vi "测试接收队列.vi"() -> ()   [LabVIEW 2015]
uses:
  <userlib>/QMH/Message Queue/Support/Enqueue Message (Single).vi
  <vilib>/Utility/error.llb/Error Cluster From Error Code.vi
  <vilib>/ErrorRing/Error Ring.xnode
  <userlib>/QMH/User Event - Stop/User Event - Stop.lvlib
  <userlib>/QMH/Message Queue/Message Queue.lvlib
panel:
  in  "表格":string[][](table)
  in  "Exit":bool
  in  "HostThread":variant
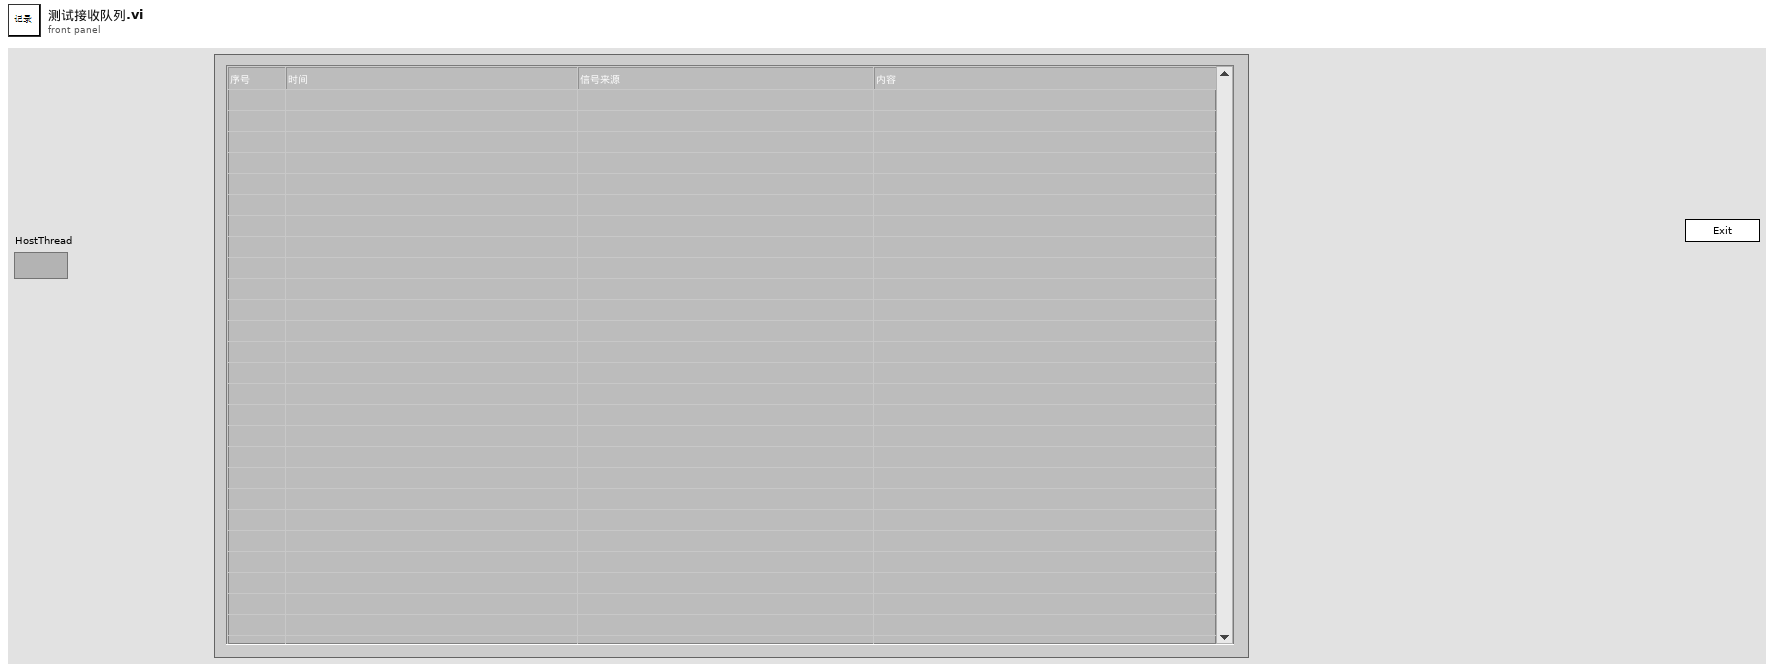
[diagram p1: front panel]
types:
  T1 = cluster{"Controls":cluster{"Exit":refnum<vi>, "表格":refnum<vi>}, "Thread":cluster{"ThisQ":string, "ThisVI":refnum<vi>, "HostQ":string, "HostRef":refnum<vi>, "SlavesQ":string[], "SlavesRef":refnum<vi>[]}, "Data":cluster{"Replace":bool}, "User":cluster{"Name":string}, "文本":string[], "计数":i32}
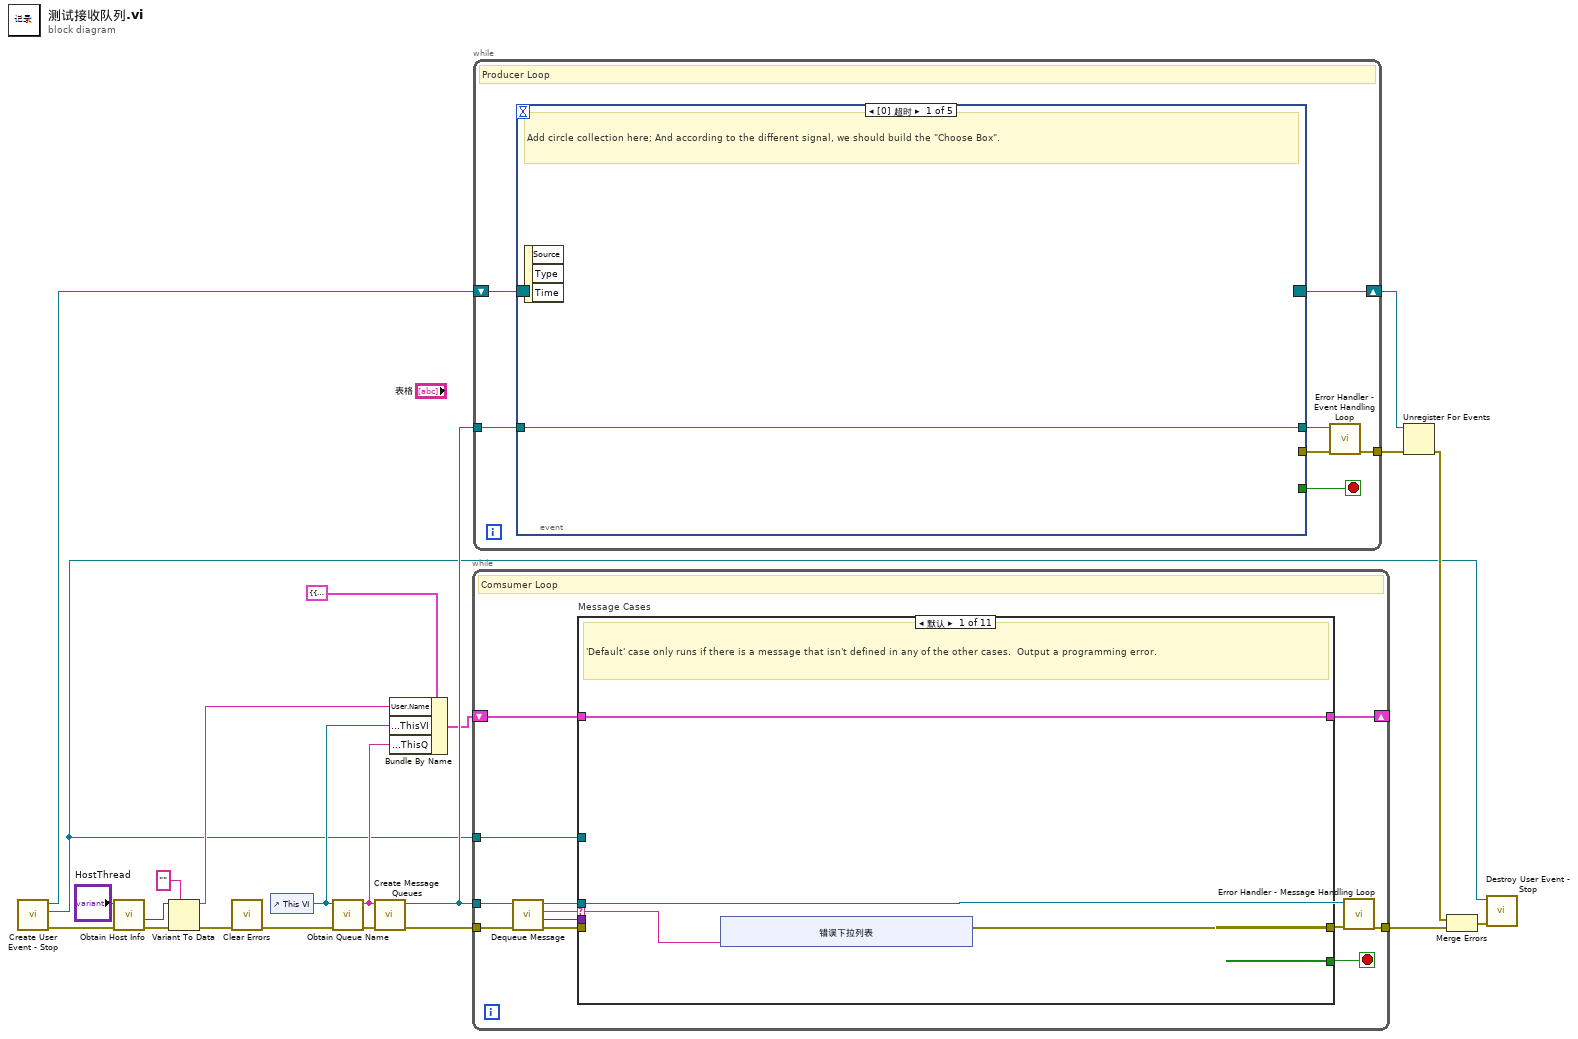
[diagram p0: block diagram]
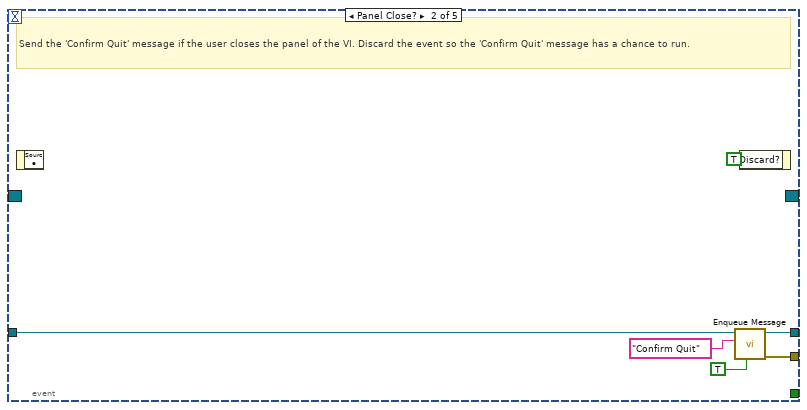
[diagram p2: hidden frame]
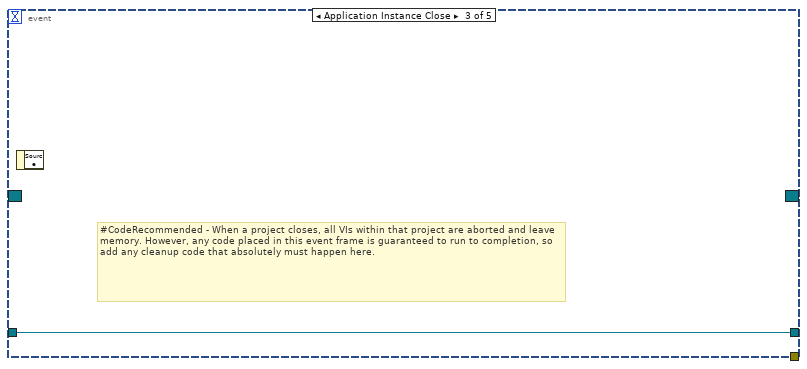
[diagram p3: hidden frame]
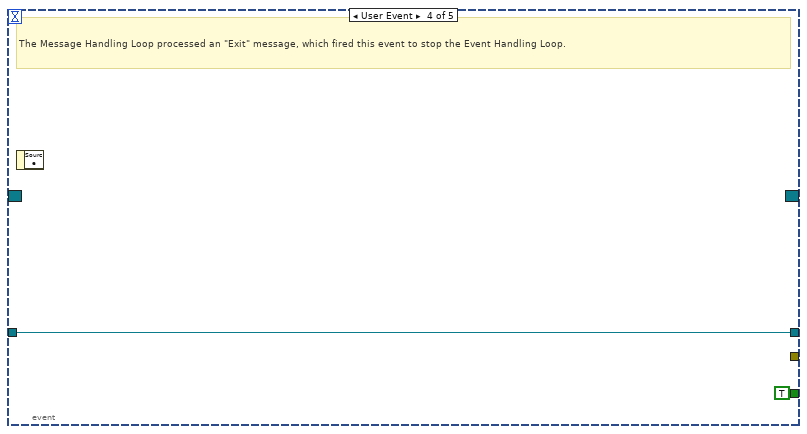
[diagram p4: hidden frame]
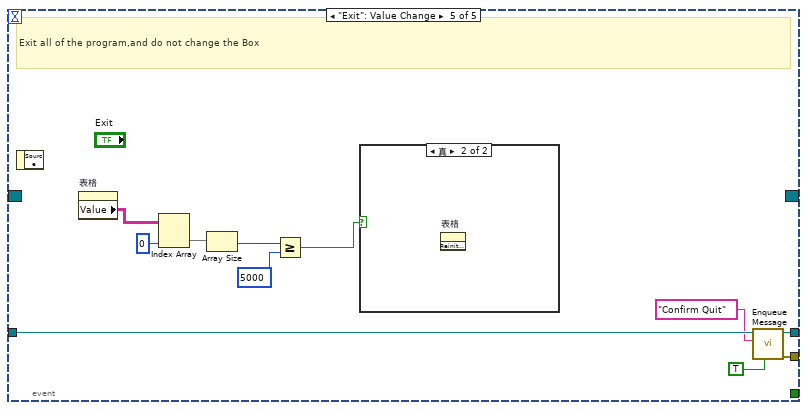
[diagram p5: hidden frame]
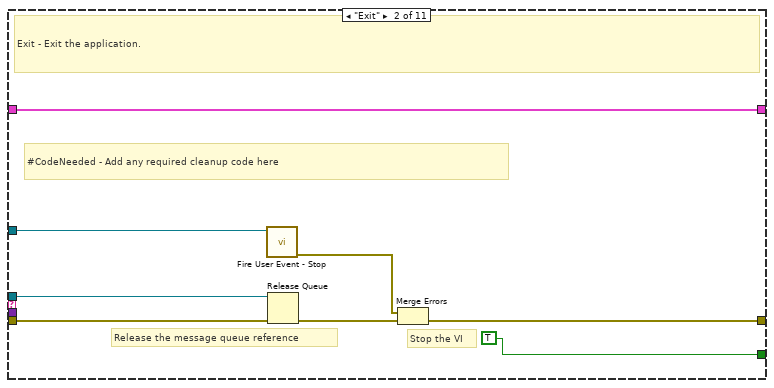
[diagram p7: hidden frame]
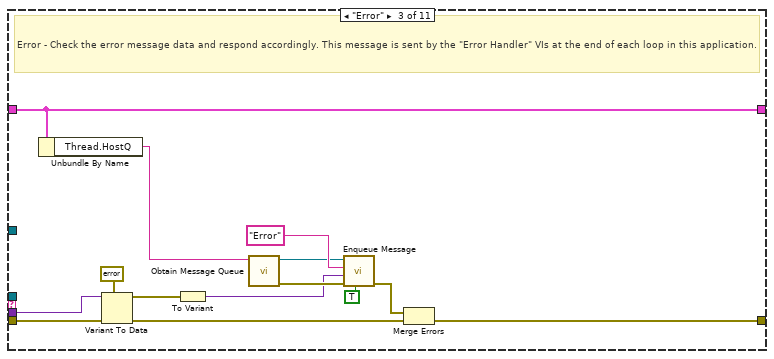
[diagram p8: hidden frame]
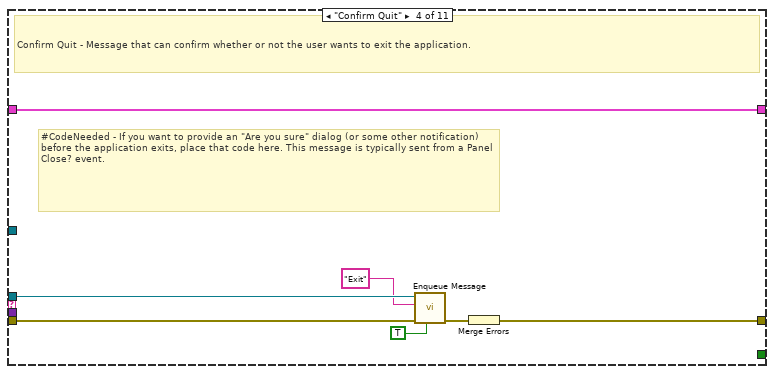
[diagram p9: hidden frame]
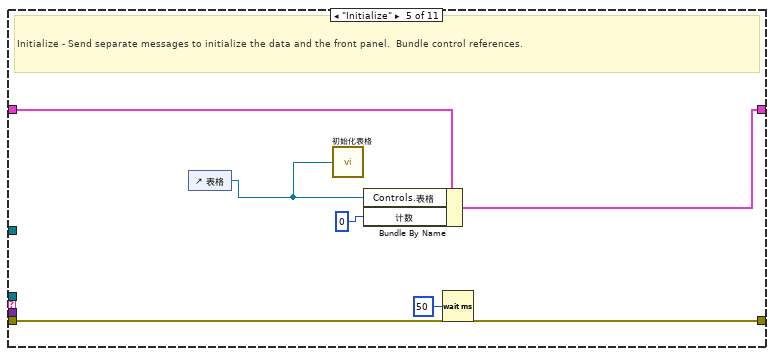
[diagram p10: hidden frame]
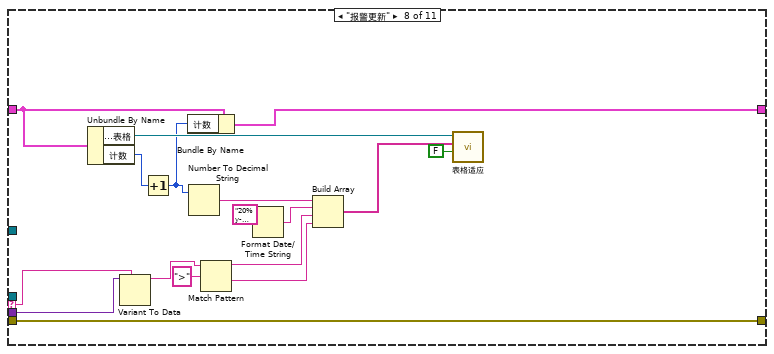
[diagram p13: hidden frame]
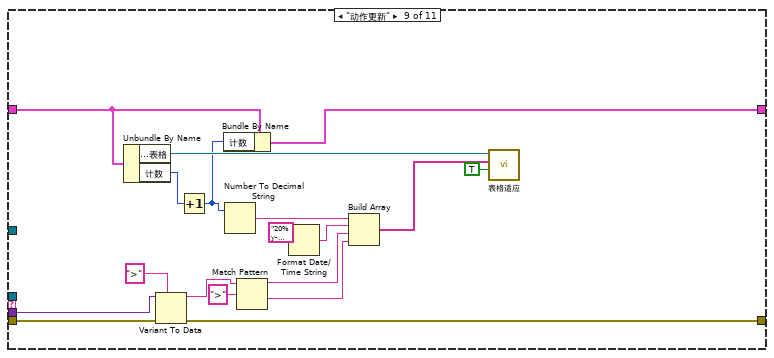
[diagram p14: hidden frame]
diagram:
  n1 = call <userlib>:"Create User Event - Stop.vi"() -> ("error out"=w14:errorcluster, "User Event - Stop"=w5:refnum<user-event>, "Stop Event Registration Refnum"=w3:refnum<event-registration>)  [unwired: 9 in]
  n2 = call <userlib>:"Obtain Host Info.vi"("error in (no error)"=w14, "HostThread"="HostThread") -> ("error out"=w17:errorcluster, "Data"=w18:variant)  [unwired: 6 in, 2 out]
  n3 = Variant To Data(error in=w17, type="", Variant=w18) -> (data=w22:string, error out=w20:errorcluster)
  n4 = call <vilib>:"Clear Errors.vi"("error in (no error)"=w20) -> ("error out"=w21:errorcluster)  [unwired: 5 in, 1 out]
  n5 = control-ref of="This VI"() -> (w12:refnum<vi>)
  n6 = call <userlib>:"Obtain Queue Name.vi"("error in (no error)"=w21, "VI Refnum"=w12) -> ("error out"=w9:errorcluster, "ViName"=w13:string)  [unwired: 8 in]
  n7 = call <userlib>:"Create Message Queues.vi"("error in (no error)"=w9, "name (unnamed)"=w13) -> ("error out"=w1:errorcluster, "QueueHandler"=w16:refnum<queue>)  [unwired: 8 in]
  n8 = Bundle By Name(cluster=T1 {"Controls"={"Exit"=refnum, "表格"=refnum}, "Thread"={"ThisQ"="", "ThisVI"=refnum, "HostQ"="", "HostRef"=refnum, "SlavesQ"=[], "SlavesRef"=[]}, "Data"={"Replace"=FALSE}, "User"={"Name"=""}, "文本"=[], "计数"=0} ("Data Cluster"), "User.Name"=w22, "Thread.ThisVI"=w12, "Thread.ThisQ"=w13) -> (w11:T1)
  n9 = while {
    tunnel: w16 -> [w26]
    shift-right: [w33] -> _
    shift-left: w11 -> [w34]
    tunnel: w5 -> [w31]
    tunnel: w1 -> [w30]
    tunnel: [w24] -> w2
    stop <- w32 stop-if-true
    # "Comsumer Loop"
    n10 = call <userlib>:"Dequeue Message.vi"("error in (no error)"=w30, "Message Queue"=w26) -> ("error out"=w29:errorcluster, "Message Data"=w27:variant, "Message"=w28:string, "dup Message Queue"=w25:refnum<queue>)  [unwired: 6 in]
    n11 = case "Message Cases" shown="默认" w28 {
      selector: w28 -> [w35 _ _ _ _ _ _ w98 _ _ _]
      tunnel: w25 -> [_ w52 _ w69 _ _ _ _ _ _ _]
      tunnel: w29 -> [_ w47 w66 w73 w79 w81 w83 w100 w117 w118 w121]
      tunnel: [w36 w48 w61 w71 w79 w81 w83 w100 w117 w118 w121] -> w23
      tunnel: w34 -> [w37 w51 w58 w72 w78 w80 w82 w86 w104 w119 w120]
      tunnel: [w37 w51 w58 w72 w77 w80 w82 w85 w105 w119 w120] -> w33
      tunnel: [_ TRUE _ _ _ _ _ _ _ _ _] -> w32
      tunnel: w27 -> [_ _ w65 _ _ _ _ w99 w103 _ _]
      tunnel: w31 -> [_ w46 _ _ _ _ _ _ _ _ _]
      frame Default {
        # "'Default' case only runs if there is a message that isn't defined in any of the other cases.  Output a programming error."
        n12 = xnode "错误下拉列表"("参数 0"=w35) -> ("错误输出"=w36:errorcluster)
      }
      frame "Exit" {
        # "Stop the VI"
        # "Release the message queue reference"
        # "#CodeNeeded - Add any required cleanup code here"
        # "Exit - Exit the application."
        n13 = call <userlib>:"Fire User Event - Stop.vi"("User Event - Stop"=w46) -> ("error out"=w45:errorcluster)  [unwired: 10 in]
        n14 = Release Queue(queue=w52, error in (no error)=w47) -> (error out=w49:errorcluster)  [unwired: 1 in, 2 out]
        n15 = Merge Errors(w45, w49) -> (w48:errorcluster)
      }
      frame "Error" {
        # "Error - Check the error message data and respond accordingly. This message is sent by the \"Error Handler\" VIs at the end of each loop in this application."
        n16 = Unbundle By Name(w58) -> ("Thread.HostQ"=w57:string)
        n17 = Variant To Data(error in=w66, type=errorcluster {"status"=FALSE, "code"=0, "source"=""} ("error constant"), Variant=w65) -> (data=w54:errorcluster, error out=w63:errorcluster)
        n18 = To Variant(anything=w54) -> (Variant=w53:variant)
        n19 = call <userlib>:"Obtain Message Queue.vi"("name (unnamed)"=w57) -> ("error out"=w56:errorcluster, "Message Queue"=w55:refnum<queue>)  [unwired: 9 in]
        n20 = call-poly <userlib>:"Enqueue Message.vi"("Priority Message? (F)"=TRUE, "error in (no error)"=w56, "Message Data"=w53, "Message"="Error", "Message Queue"=w55) -> ("error out"=w62:errorcluster)  [unwired: 5 in, 1 out]
        n21 = Merge Errors(w62, w63) -> (w61:errorcluster)
      }
      frame "Confirm Quit" {
        # "#CodeNeeded - If you want to provide an \"Are you sure\" dialog (or some other notification) before the application exits, place that code here. This message is typically sent from a Panel Close? event."
        # "Confirm Quit - Message that can confirm whether or not the user wants to exit the application."
        n22 = call-poly <userlib>:"Enqueue Message.vi"("Priority Message? (F)"=TRUE, "error in (no error)"=w73, "Message"="Exit", "Message Queue"=w69) -> ("error out"=w70:errorcluster)  [unwired: 6 in, 1 out]
        n23 = Merge Errors(w70) -> (w71:errorcluster)
      }
      frame "Initialize" {
        # "Initialize - Send separate messages to initialize the data and the front panel.  Bundle control references."
        n24 = control-ref of="表格"() -> (w74:refnum<vi>)
        n25 = call "初始化表格.vi"("引用"=w74) -> ()
        n26 = Bundle By Name(cluster=w78, "Controls.表格"=w74, "计数"=0) -> (w77:T1)
        n27 = Wait (ms)(milliseconds to wait=u32 50 ("等待时间（毫秒）")) -> ()  [unwired: 1 out]
      }
      frame "<-------UI-------->" {
      }
      frame "<------Core------>" {
      }
      frame "报警更新" {
        n28 = Unbundle By Name(w86) -> ("Controls.表格"=w90:refnum<vi>, "计数"=w96:i32)
        n29 = Variant To Data(type=w98, Variant=w99) -> (data=w97:string)  [unwired: 1 in, 1 out]
        n30 = Increment(x=w96) -> (x+1=w84:i32)
        n31 = Bundle By Name(cluster=w86, "计数"=w84) -> (w85:T1)
        n32 = Number To Decimal String(number=w84) -> (decimal integer string=w95:string)  [unwired: 1 in]
        n33 = Match Pattern(string=w97, regular expression=">" ("正则表达式")) -> (before substring=w92:string, after substring=w91:string)  [unwired: 1 in, 2 out]
        n34 = Format Date/Time String(time format string (%c)="20%y-%m-%d  %H：%M：%S" ("时间格式字符串(%c)")) -> (date/time string=w93:string)  [unwired: 2 in]
        n35 = Build Array(w95, w93, w92, w91) -> (w89:string[])
        n36 = call "表格适应.vi"("Red-F"=FALSE, "new"=w89, "表格in"=w90) -> ()  [unwired: 9 in]
      }
      frame "动作更新" {
        n37 = Unbundle By Name(w104) -> ("Controls.表格"=w110:refnum<vi>, "计数"=w116:i32)
        n38 = Variant To Data(type=">" ("正则表达式"), Variant=w103) -> (data=w101:string)  [unwired: 1 in, 1 out]
        n39 = Increment(x=w116) -> (x+1=w106:i32)
        n40 = Bundle By Name(cluster=w104, "计数"=w106) -> (w105:T1)
        n41 = Number To Decimal String(number=w106) -> (decimal integer string=w115:string)  [unwired: 1 in]
        n42 = Match Pattern(string=w101, regular expression=">" ("正则表达式")) -> (before substring=w112:string, after substring=w111:string)  [unwired: 1 in, 2 out]
        n43 = Format Date/Time String(time format string (%c)="20%y-%m-%d  %H：%M：%S" ("时间格式字符串(%c)")) -> (date/time string=w113:string)  [unwired: 2 in]
        n44 = Build Array(w115, w113, w112, w111) -> (w109:string[])
        n45 = call "表格适应.vi"("Red-F"=TRUE, "new"=w109, "表格in"=w110) -> ()  [unwired: 9 in]
      }
      frame "Core_InitializeRef" {
        # "Initialize control references. For there is not enough space to locate all the control references, separate the codes into 2 messages"
      }
      frame "<---Operation--->" {
      }
    }
    n46 = call <userlib>:"Error Handler - Message Handling Loop.vi"("error in (no error)"=w23, "Message Queue"=w25) -> ("dup error in"=w24:errorcluster)  [unwired: 8 in, 1 out]
  }
  n47 = while {
    tunnel: w16 -> [w128]
    shift-right: [w126] -> w7
    shift-left: w3 -> [w127]
    tunnel: [w122] -> w8
    stop <- w124 stop-if-true
    # "Producer Loop"
    n48 = event shown="[0] 超时" {
      selector: w127 -> [_ _ _ _ _]
      dyn-events: [_ _ _ _ _] -> w126
      timeout: _ -> [_ _ _ _ _]
      tunnel: [_ _ _ TRUE ("Discard?") _] -> w124
      tunnel: w128 -> [w129 w134 w136 w138 w149]
      tunnel: [_ w133 _ _ w147] -> w125
      tunnel: [w129 w132 w136 w138 w148] -> w123
      event Timeout {
        # "Add circle collection here; And according to the different signal, we should build the \"Choose Box\"."
        n49 = event-data() -> ()  [unwired: 1 in, 3 out]
      }
      event Panel Close? {
        # "Send the 'Confirm Quit' message if the user closes the panel of the VI. Discard the event so the 'Confirm Quit' message has a chance to run."
        n50 = event-data() -> ()  [unwired: 1 in, 1 out]
        n51 = call-poly <userlib>:"Enqueue Message.vi"("Priority Message? (F)"=TRUE, "Message"="Confirm Quit", "Message Queue"=w134) -> ("error out"=w133:errorcluster, "dup Message Queue"=w132:refnum<queue>)  [unwired: 7 in]
        n52 = event-data("Discard?"=TRUE) -> ()  [unwired: 1 in, 1 out]
      }
      event Application Instance Close {
        # "#CodeRecommended - When a project closes, all VIs within that project are aborted and leave memory. However, any code placed in this event frame is guaranteed to run to completion, so add any cleanup code that absolutely must happen here."
        n53 = event-data() -> ()  [unwired: 1 in, 1 out]
      }
      event User Event {
        # "The Message Handling Loop processed an \"Exit\" message, which fired this event to stop the Event Handling Loop."
        n54 = event-data() -> ()  [unwired: 1 in, 1 out]
      }
      event "Exit": Value Change {
        # "Exit all of the program,and do not change the Box"
        n55 = event-data() -> ()  [unwired: 1 in, 1 out]
        n56 = property on="表格" class="Tbl (严格)"() -> ("Value"=w142:string[][])  [unwired: 2 in, 2 out]
        n57 = Index Array(array=w142, index (col)=0 ("禁用的索引 (列)")) -> (element=w143:string[])  [unwired: 1 in]
        n58 = Array Size(array=w143) -> (size(s)=w141:i32)
        n59 = Greater Or Equal?(x=w141, y=5000) -> (x >= y?=w139:bool)
        n60 = case shown="真" w139 {
          frame False {
          }
          frame True {
            n61 = invoke on="表格" class="Tbl (严格)" method="Reinit To Default"() -> ()  [unwired: 3 in, 3 out]
          }
        }
        n62 = call-poly <userlib>:"Enqueue Message.vi"("Priority Message? (F)"=TRUE, "Message"="Confirm Quit", "Message Queue"=w149) -> ("error out"=w147:errorcluster, "dup Message Queue"=w148:refnum<queue>)  [unwired: 7 in]
      }
    }
    n63 = call <userlib>:"Error Handler - Event Handling Loop.vi"("error in (no error)"=w125, "Message Queue"=w123) -> ("dup error in"=w122:errorcluster)  [unwired: 8 in, 1 out]
  }
  n64 = Unregister For Events(event registration refnum=w7, error in=w8) -> (error out=w6:errorcluster)
  n65 = Merge Errors(w6, w2) -> (w4:errorcluster)
  n66 = call <userlib>:"Destroy User Event - Stop.vi"("error in (no error)"=w4, "User Event - Stop"=w5) -> ()  [unwired: 9 in, 1 out]
